vi "SetRoughGainandFineGain.vi"(8 "error in (no error)":errorcluster, 10 "reference":refnum<k7>, 11 "IN":T1={"step name 1"="", "updata 2"="1000", "limitdata 3"="", "load vi name 4"="", "parameter 5"=""}) -> (0 "error out":errorcluster, 2 "reference out":refnum<k7>, 3 "Cluster":T2)   [LabVIEW 2013]
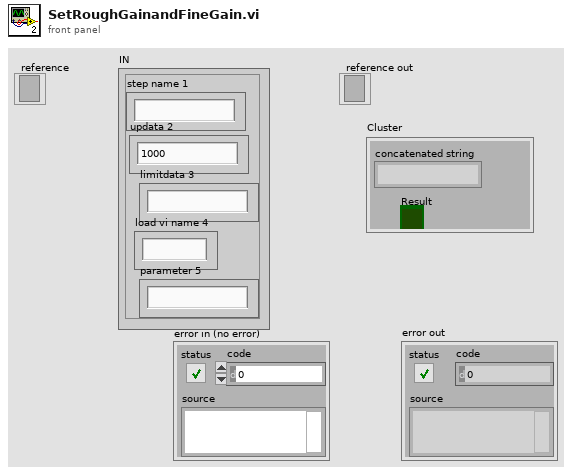
[diagram p1: front panel]
types:
  T1 = cluster{"step name 1":string, "updata 2":string, "limitdata 3":string, "load vi name 4":string, "parameter 5":string}
  T2 = cluster{"concatenated string":string, "Result":bool}
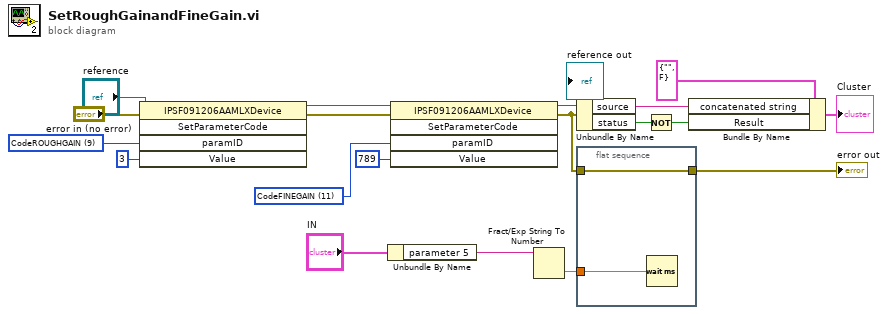
[diagram p0: block diagram]
diagram:
  w9 = 11 items=["CodeTC2ND"=1, "CodeTC1ST"=2, "CodeOFFDRIFT"=3, "CodeFILTCODE"=4, "CodeDCDEF"=5, "CodeSWITCH"=6, "CodeCLAMP"=7, "CodeOUTMODE"=8, "CodeROUGHGAIN"=9, "CodeOUTSLOPE"=10, "CodeFINEGAIN"=11, "CodeDIAGINFAULT"=12, "CodeREFEDGE"=13, "CodeYA"=14, "CodeXA"=15, "CodeCSTID"=16, "CodeMLXID1"=17, "CodeMLXID2"=18, "CodeMLXID3"=19, "CodeCRC10"=20, "CodeRATIODIS"=21, "CodeTC2NDHOT"=22, "CodeTC2NDCOLD"=23, "CodeOFFDRIFTHOT"=24, "CodeOFFDRIFTCOLD"=25, "CodeCLAMPLOW"=26, "CodeCLAMPHIGH"=27, "CodePLATEPOL"=28, "CodeDSPMODE"=104, "CodeTHERMOSLOPE"=106, "CodeTHERMOOFF"=107, "CodeDeltaTC1ST_RGP1"=29, "CodeDeltaTC1ST_RGM1"=30, "CodeDeltaOD_RGP1"=31, "CodeDeltaOD_RGM1"=32, "CodeOPTIONCODE"=33, "CodeLOTNUMBER"=34] ("paramID")
  w10 = 9 items=["CodeTC2ND"=1, "CodeTC1ST"=2, "CodeOFFDRIFT"=3, "CodeFILTCODE"=4, "CodeDCDEF"=5, "CodeSWITCH"=6, "CodeCLAMP"=7, "CodeOUTMODE"=8, "CodeROUGHGAIN"=9, "CodeOUTSLOPE"=10, "CodeFINEGAIN"=11, "CodeDIAGINFAULT"=12, "CodeREFEDGE"=13, "CodeYA"=14, "CodeXA"=15, "CodeCSTID"=16, "CodeMLXID1"=17, "CodeMLXID2"=18, "CodeMLXID3"=19, "CodeCRC10"=20, "CodeRATIODIS"=21, "CodeTC2NDHOT"=22, "CodeTC2NDCOLD"=23, "CodeOFFDRIFTHOT"=24, "CodeOFFDRIFTCOLD"=25, "CodeCLAMPLOW"=26, "CodeCLAMPHIGH"=27, "CodePLATEPOL"=28, "CodeDSPMODE"=104, "CodeTHERMOSLOPE"=106, "CodeTHERMOOFF"=107, "CodeDeltaTC1ST_RGP1"=29, "CodeDeltaTC1ST_RGM1"=30, "CodeDeltaOD_RGP1"=31, "CodeDeltaOD_RGM1"=32, "CodeOPTIONCODE"=33, "CodeLOTNUMBER"=34] ("paramID")
  n1 = invoke class="IPSF091206AAMLXDevice" method="SetParameterCode"(reference="reference", error in="error in (no error)", "paramID"=w10, "Value"=3) -> (reference out=w13:refnum<k7>, error out=w12:errorcluster)  [unwired: 1 in, 3 out]
  n2 = Unbundle By Name("IN") -> ("parameter 5"=w15:string)
  n3 = invoke class="IPSF091206AAMLXDevice" method="SetParameterCode"(reference=w13, error in=w12, "paramID"=w9, "Value"=789) -> (reference out=→"reference out":refnum<k7>, error out=w6:errorcluster)  [unwired: 1 in, 3 out]
  n4 = Fract/Exp String To Number(string=w15) -> (number=w16:dbl)  [unwired: 3 in, 1 out]
  n5 = Unbundle By Name(w6) -> ("source"=w3:string, "status"=w5:bool)
  n6 = flat-sequence {
    tunnel: w6 -> [w20]
    tunnel: w16 -> [w21]
    tunnel: [w20] -> w14
    frame #0 {
      n7 = Wait (ms)(milliseconds to wait=w21) -> ()  [unwired: 1 out]
    }
  }
  n8 = Not(x=w5) -> (.not. x?=w4:bool)
  n9 = Bundle By Name(cluster=T2 {"concatenated string"="", "Result"=FALSE} ("Cluster"), "concatenated string"=w3, "Result"=w4) -> (→"Cluster":T2)
  "error out" <- w14
